vi "Set Debugging Level.vi"(8 "error in (no error)":errorcluster, 11 "Debug Level in":T1=enum."DEBUG") -> (0 "error out":errorcluster)   [LabVIEW 2020, in "LV Log.lvlib"]
uses:
  LV Log.lvlib
  Type Defs/Debug Level.ctl
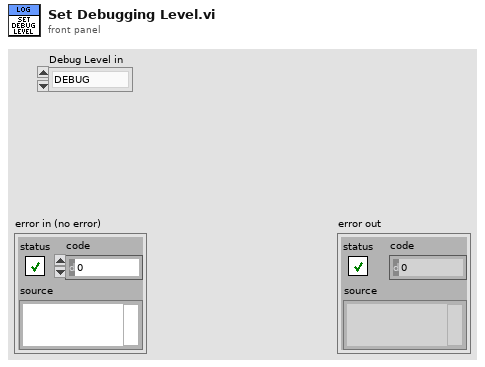
[diagram p1: front panel]
types:
  T1 = typedef "LV Log.lvlib/Debug Level.ctl" = enum16{"DEFAULT", "DEBUG", "INFO", "WARN", "ERROR", "FATAL"}
  T2 = enum16{"Init", "Get Logger", "Register Sink", "Set Global Debug Level", "Get Sinks"}
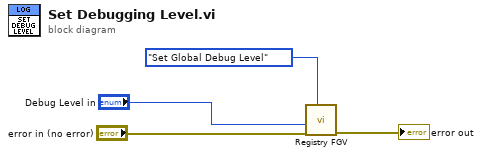
[diagram p0: block diagram]
diagram:
  n1 = call "Registry FGV.vi"("State (Get Logger)"=T2."Set Global Debug Level", "error in (no error)"="error in (no error)", "Debug Level in"="Debug Level in") -> ("error out"=→"error out":errorcluster)  [unwired: 5 in, 3 out]
